vi "time since midnight.vi"(0 "seconds since 1Jan1904":dbl format="%.2f") -> (1 "seconds":u32 format="%<%H:%M:%S%0u>t", 2 "Days":dbl format="%.2f")   [LabVIEW 2015]
doc: "Seconds since the beginning of today based on local time."
panel:
  in  "date time rec":T1
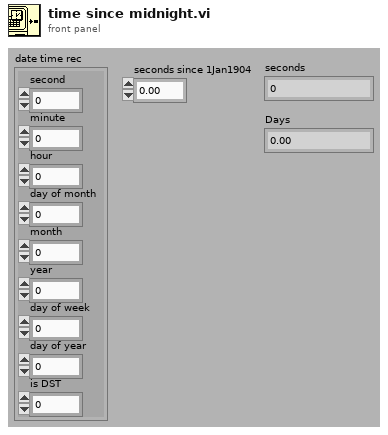
[diagram p1: front panel]
types:
  T1 = cluster{"second":i32, "minute":i32, "hour":i32, "day of month":i32, "month":i32, "year":i32, "day of week":i32, "day of year":i32, "is DST":i32}
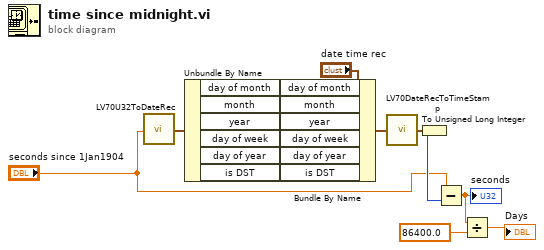
[diagram p0: block diagram]
diagram:
  n1 = call <vilib>:"LV70U32ToDateRec.vi"("Time"="seconds since 1Jan1904") -> ("date time rec"=w15:T1)
  n2 = Unbundle By Name(w15) -> ("day of month"=w12:i32, "month"=w11:i32, "year"=w10:i32, "day of week"=w9:i32, "day of year"=w8:i32, "is DST"=w7:i32)
  n3 = Bundle By Name(cluster="date time rec", "day of month"=w12, "month"=w11, "year"=w10, "day of week"=w9, "day of year"=w8, "is DST"=w7) -> (w14:T1)
  n4 = call <vilib>:"LV70DateRecToTimeStamp.vi"("date time rec"=w14) -> ("Time Stamp"=w1:timestamp)
  n5 = To Unsigned Long Integer(number=w1) -> (unsigned 32bit integer=w6:u32)
  n6 = Subtract(x="seconds since 1Jan1904", y=w6) -> (x-y=w4:dbl)
  "seconds" <- w4
  n7 = Divide(x=w4, y=86400.0) -> (x/y=→"Days":dbl)
